vi "Get Error (ID).vi"(8 "error in (no error)":errorcluster, 10 "ID":string, 11 "error list <owner>":variant) -> (0 "error out":errorcluster, 1 "found?":bool, 2 "error":T1, 3 "error list <owner> dup":variant, 4 "attributes":string[](array[string]))   [LabVIEW 2017]
uses:
  Error File Management/Controls/NI Error.ctl
  Attributes.vi
  Error File Management/Error File Management.lvlib
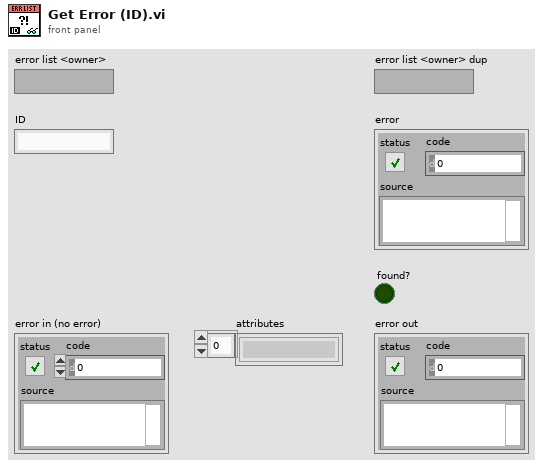
[diagram p1: front panel]
types:
  T1 = typedef "Error File Management.lvlib/NI Error.ctl" = errorcluster
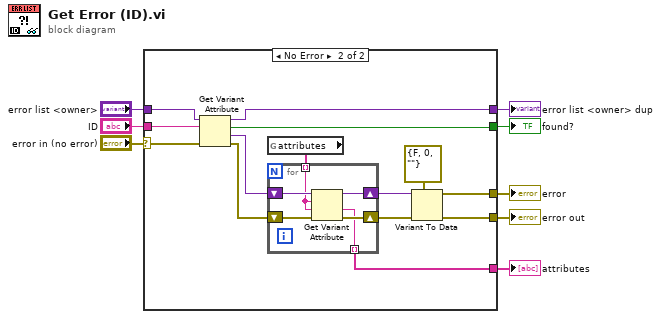
[diagram p0: block diagram]
diagram:
  n1 = case shown="No Error" "error in (no error)" {
    selector: "error in (no error)" -> [w10 w20]
    tunnel: "error list <owner>" -> [w9 w23]
    tunnel: [w9 w24] -> w7
    tunnel: [w10 w18] -> w5
    tunnel: "ID" -> [_ w21]
    tunnel: [_ w17] -> w3
    tunnel: [_ w16] -> w2
    tunnel: [_ w11] -> w1
    frame Error {
    }
    frame No Error {
      n2 = Get Variant Attribute(Variant=w23, name=w21, error in=w20) -> (duplicate Variant=w24:variant, found=w16:bool, value=w22:variant, error out=w19:errorcluster)  [unwired: 1 in]
      n3 = global read "Attributes.vi" "attributes"() -> (w12:string[])
      n4 = for {
        tunnel: [w25] -> w11 mode=indexing
        shift-right: [w28] -> w14
        shift-left: w22 -> [w30]
        shift-right: [w27] -> w13
        shift-left: w19 -> [w29]
        tunnel: w12 -> [w26] mode=indexing
        n5 = Get Variant Attribute(Variant=w30, name=w26, default value (empty Variant)=w26, error in=w29) -> (duplicate Variant=w28:variant, value=w25:string, error out=w27:errorcluster)  [unwired: 1 out]
      }
      n6 = Variant To Data(error in=w13, type=T1 {"status"=FALSE, "code"=0, "source"=""} ("error"), Variant=w14) -> (data=w17:T1, error out=w18:errorcluster)
    }
  }
  "error list <owner> dup" <- w7
  "error out" <- w5
  "error" <- w3
  "found?" <- w2
  "attributes" <- w1
